vi "TCP Generic Listener.vi"(0 "net address":u32, 5 "port":u16, 11 "error in (no error)":errorcluster) -> (4 "connection ID":refnum<k5>, 8 "Connected?":bool, 15 "error out":errorcluster)   [LabVIEW 2020]
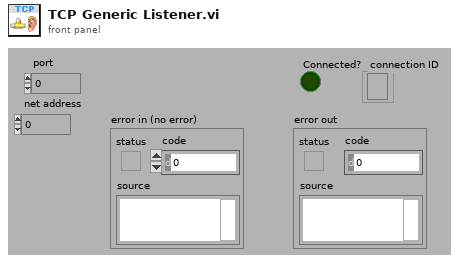
[diagram p1: front panel]
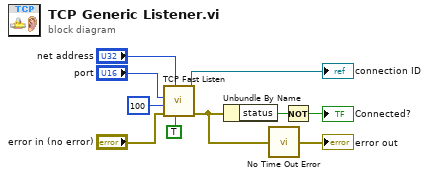
[diagram p0: block diagram]
diagram:
  n1 = call "TCP Fast Listen.vi"("TCP_NODELAY (true)"=TRUE, "net address"="net address", "error in (no error)"="error in (no error)", "timeout ms (wait forever: -1)"=100, "port"="port") -> ("error out"=w8:errorcluster, "connection ID"=→"connection ID":refnum<k5>)  [unwired: 3 in, 2 out]
  n2 = Unbundle By Name(w8) -> ("status"=w9:bool)
  n3 = call "No Time Out Error.vi"("error in"=w8) -> ("error out"=→"error out":errorcluster)  [unwired: 14 in]
  n4 = Not(x=w9) -> (.not. x?=→"Connected?":bool)
